vi "Setup subWorker - SDAQ.vi"(8 "error in":errorcluster, 11 "UserInterface in":refnum<class "UserInterface.lvclass">) -> (0 "error out":errorcluster, 3 "UserInterface out":refnum<class "UserInterface.lvclass">)   [LabVIEW 2017, in "UserInterface.lvclass"]
doc: "<b>Note: Do not change the code in this VI!</b>\nThis VI performs a setup of all the statically-linked subWorkers that belong to the Worker that calls this VI. This VI is created automatically by the 'Create/Add Worker' tool and must be called <b>before</b> any statically linked subWorkers are called."
uses:
  UserInterface.lvclass
  SimulationDaq/SimulationDaq.lvclass
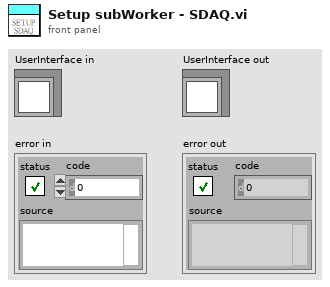
[diagram p1: front panel]
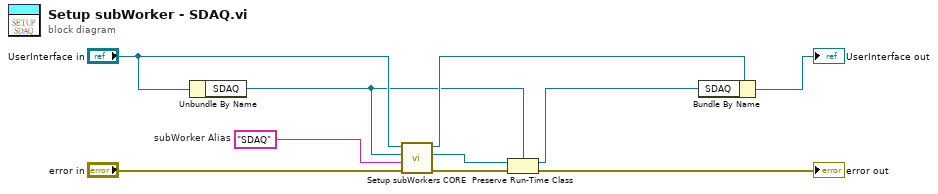
[diagram p0: block diagram]
diagram:
  w6 = "SDAQ"  # subWorker Alias
  n1 = Unbundle By Name("UserInterface in") -> ("SDAQ"=w3:refnum<class "SimulationDaq.lvclass">)
  n2 = call-dynamic "Setup subWorkers CORE.vi"("error in"="error in", "subWorker Alias"=w6, "subWorker"=w3, "Worker"="UserInterface in") -> ("error out"=w5:errorcluster, "subWorker out"=w1:refnum<class "Worker.lvclass">, "Worker out"=w8:refnum<class "UserInterface.lvclass">)  [unwired: 5 in]
  n3 = Preserve Run-Time Class(object in=w1, error in=w5, 2:w3) -> (object out=w2:refnum<class "SimulationDaq.lvclass">, error out=→"error out":errorcluster)
  n4 = Bundle By Name(cluster=w8, "SDAQ"=w2) -> (→"UserInterface out":refnum<class "UserInterface.lvclass">)
